vi "INI-ListStringValues.vi"(8 "error in (no error)":errorcluster, 10 "Session(\"\" for all)":string, 11 "configuration file path":path) -> (0 "error out":errorcluster, 1 "value":string[](array[string]), 2 "Keys":string[](array[string]))   [LabVIEW 2017, in "INI++.lvlib"]
uses:
  INI++.lvlib
  <vilib>/Utility/config.llb/Read Key (String).vi
  <vilib>/Utility/config.llb/NI_LVConfig.lvlib
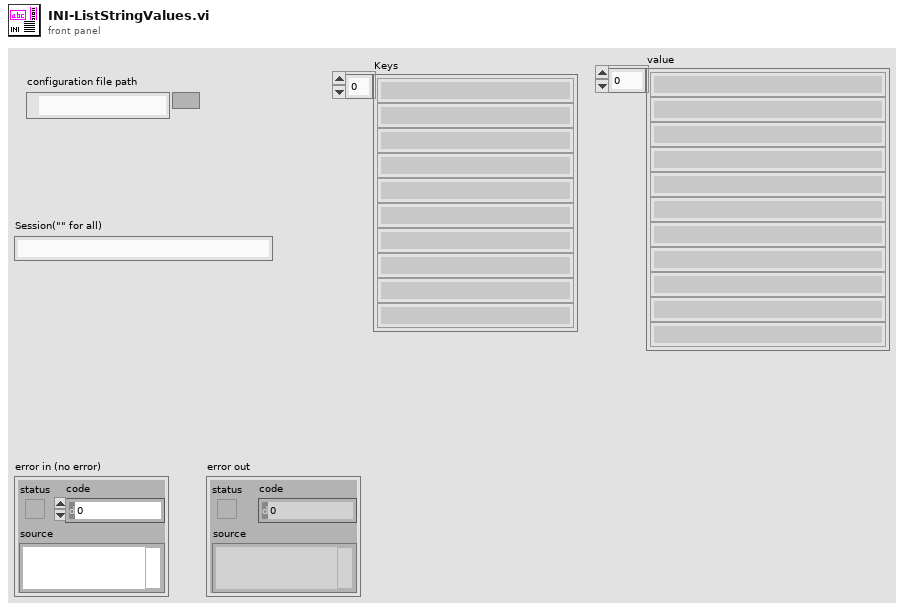
[diagram p1: front panel]
types:
  T1 = typedef "NI_LVConfig.lvlib/Config Data RefNum.ctl" = refnum<k1>
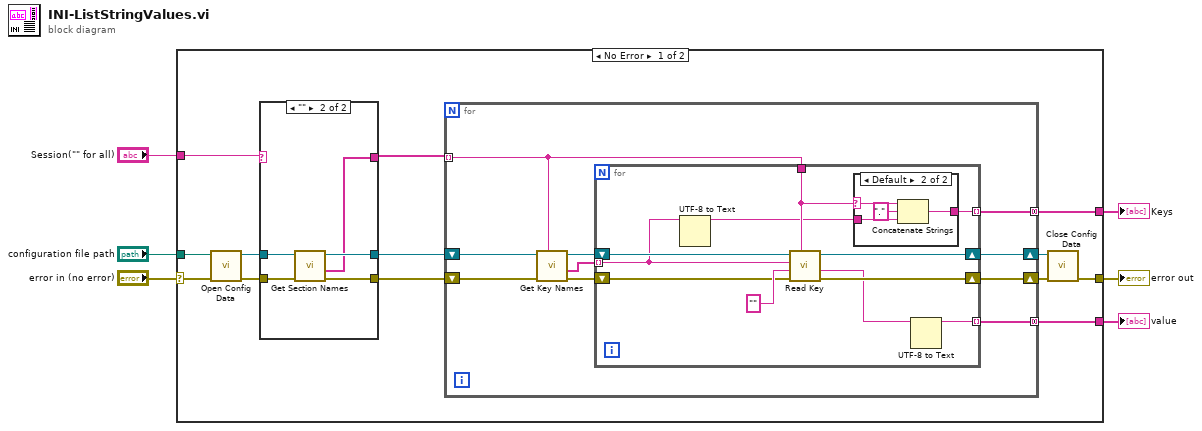
[diagram p0: block diagram]
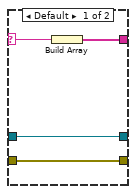
[diagram p2: hidden frame]
diagram:
  n1 = case shown="No Error" "error in (no error)" {
    selector: "error in (no error)" -> [w14 w55]
    tunnel: [w13 _] -> w5
    tunnel: [w11 w55] -> w4
    tunnel: "Session(\"\" for all)" -> [w9 _]
    tunnel: [w8 _] -> w2
    tunnel: "configuration file path" -> [w7 _]
    frame No Error {
      n2 = call <vilib>:"Open Config Data.vi"("error in (no error)"=w14, "configuration file path"=w7) -> ("error out"=w18:errorcluster, "refnum"=w19:T1)  [unwired: 7 in, 1 out]
      n3 = case shown="\"\"" w9 {
        selector: w9 -> [w23 _]
        tunnel: w19 -> [w21 w28]
        tunnel: w18 -> [w20 w27]
        tunnel: [w21 w26] -> w17
        tunnel: [w20 w25] -> w16
        tunnel: [w22 w24] -> w15
        frame Default {
          n4 = Build Array(w23) -> (w22:string[])
        }
        frame "" {
          n5 = call <vilib>:"Get Section Names.vi"("error in (no error)"=w27, "refnum"=w28) -> ("error out"=w25:errorcluster, "section names"=w24:string[], "refnum out"=w26:T1)  [unwired: 7 in]
        }
      }
      n6 = for {
        tunnel: w15 -> [w30] mode=indexing
        tunnel: [w36] -> w13 mode=concatenating
        shift-right: [w35] -> w12
        shift-left: w17 -> [w38]
        shift-right: [w34] -> w10
        shift-left: w16 -> [w37]
        tunnel: [w29] -> w8 mode=concatenating
        n7 = call <vilib>:"Get Key Names.vi"("section"=w30, "error in (no error)"=w37, "refnum"=w38) -> ("error out"=w32:errorcluster, "key names"=w31:string[], "refnum out"=w33:T1)  [unwired: 5 in, 1 out]
        n8 = for {
          tunnel: [w39] -> w36 mode=indexing
          shift-right: [w49] -> w35
          shift-left: w33 -> [w46]
          shift-right: [w48] -> w34
          shift-left: w32 -> [w45]
          tunnel: w31 -> [w42] mode=indexing
          tunnel: w30 -> [w44]
          tunnel: [w43] -> w29 mode=indexing
          n9 = UTF-8 to Text(11:w42) -> (3:w41:string)  [unwired: 2 in, 1 out]
          n10 = call-poly <vilib>:"Read Key.vi"("section"=w44, "error in (no error)"=w45, "default value"="", "key"=w42, "refnum"=w46) -> ("error out"=w48:errorcluster, "value"=w40:string, "refnum out"=w49:T1)  [unwired: 3 in, 1 out]
          n11 = case shown="Default" w44 {
            selector: w44 -> [_ w54]
            tunnel: w41 -> [w50 w52]
            tunnel: [w50 w51] -> w43
            frame "apt" {
            }
            frame Default {
              n12 = Concatenate Strings(w54, "." ("string"), w52) -> (w51:string)
            }
          }
          n13 = UTF-8 to Text(11:w40) -> (3:w39:string)  [unwired: 2 in, 1 out]
        }
      }
      n14 = call <vilib>:"Close Config Data.vi"("error in (no error)"=w10, "refnum"=w12) -> ("error out"=w11:errorcluster)  [unwired: 8 in, 1 out]
    }
    frame Error {
    }
  }
  "error out" <- w4
  "value" <- w5
  "Keys" <- w2
